vi "LEBITVacuum.Safety.vi"(0 "i ref in":refnum<vi>, 2 "Nickname":string[](array[string]), 4 "Nickname":string, 5 "error IO":errorcluster) -> (14 "i ref out":refnum<vi>, 19 "error out":errorcluster)   [LabVIEW 2012, in "LEBITVacuum.lvlib"]
uses:
  LEBITVacuum.lvlib
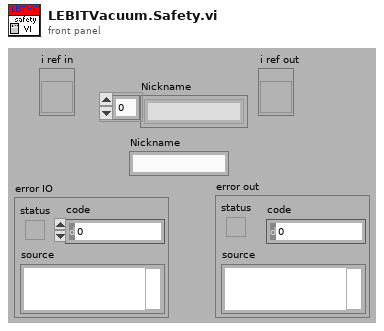
[diagram p1: front panel]
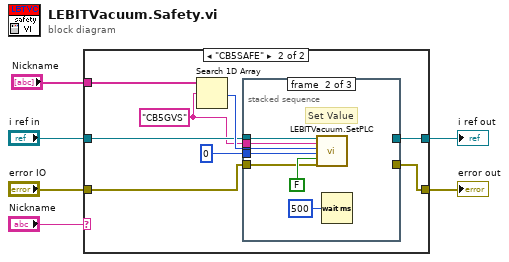
[diagram p0: block diagram]
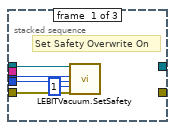
[diagram p3: hidden frame]
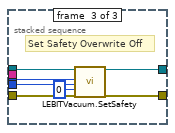
[diagram p4: hidden frame]
diagram:
  n1 = case shown="\"CB5SAFE\"" "Nickname" {
    tunnel: "i ref in" -> [w8 w11]
    tunnel: "error IO" -> [w7 w14]
    tunnel: [w8 w16] -> w3
    tunnel: [w7 w15] -> w2
    tunnel: "Nickname" -> [_ w9]
    frame Default {
    }
    frame "CB5SAFE" {
      w10 = "CB5GVS" ("element")
      n2 = Search 1D Array(1D array=w9, element=w10) -> (index of element=w12:i32)  [unwired: 1 in]
      n3 = stacked-sequence {
        tunnel: w14 -> [w21 w24 w31]
        tunnel: w12 -> [w20 w26 w33]
        tunnel: w11 -> [w19 w27 w34]
        tunnel: [_ _ w30] -> w16
        tunnel: [_ _ w29] -> w15
        tunnel: i16 0 ("Value") -> [w18 w25 w32]
        tunnel: w10 -> [_ w22 _]
        frame #0 {
          # "Set Safety Overwrite On"
          n4 = call "LEBITVacuum.SetSafety.vi"("i ref in"=w19, "index of element"=w20, "Set Value"=w18, "Safety Value"=i16 1, "error IO"=w21) -> ()  [unwired: 13 in, 2 out]
        }
        frame #1 {
          # "Set Value"
          n5 = call "LEBITVacuum.SetPLC.vi"("i ref in"=w27, "CommandName"=w22, "index of element"=w26, "Value"=w25, "log?"=FALSE, "error IO"=w24) -> ()  [unwired: 12 in, 2 out]
          n6 = Wait (ms)(milliseconds to wait=u32 500) -> ()  [unwired: 1 out]
        }
        frame #2 {
          # "Set Safety Overwrite Off"
          n7 = call "LEBITVacuum.SetSafety.vi"("i ref in"=w34, "index of element"=w33, "Set Value"=w32, "Safety Value"=i16 0, "error IO"=w31) -> ("i ref out"=w30:refnum<vi>, "error out"=w29:errorcluster)  [unwired: 13 in]
        }
      }
    }
  }
  "i ref out" <- w3
  "error out" <- w2
